vi "hidSPD Get Ready From Reports.vi"(10 "spd Reports in":T1[](array[typedef])) -> (2 "Ready":bool[](array[boolean]))   [LabVIEW 2018, in "hidSPDLibForLabView.lvlib"]
uses:
  hidSPDLibForLabView.lvlib
  hidSPD Controls/hidSPD Simple Report.ctl
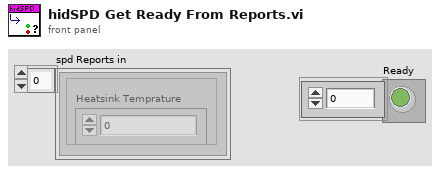
[diagram p1: front panel]
types:
  T1 = typedef "hidSPDLibForLabView.lvlib/hidSPD Simple Report.ctl" = cluster{"Heatsink Temprature":sgl, "Diod Temprature":sgl, "TEC-voltage":sgl, "Diod Bias":sgl, "RF Power":sgl, "Thermal used":sgl, "hv bias used":sgl, "hv code used":u16, "strobe code used":u16, "SPD number":u8, "SPD ready":u8}
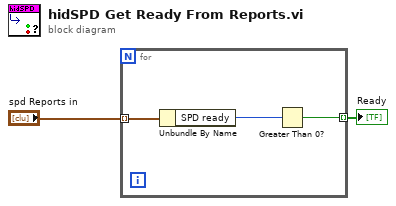
[diagram p0: block diagram]
diagram:
  n1 = for {
    tunnel: "spd Reports in" -> [w5] mode=indexing
    tunnel: [w4] -> w1 mode=indexing
    n2 = Unbundle By Name(w5) -> ("SPD ready"=w3:u8)
    n3 = Greater Than 0?(x=w3) -> (x > 0?=w4:bool)
  }
  "Ready" <- w1
